vi "Get Timestamp s.vi"(9 "error in":errorcluster) -> (1 "error out":errorcluster, 2 "Timestamp":u64 format="%d ms")   [LabVIEW 2025, in "NET based Helpers.lvlib"]
uses:
  NET based Helpers.lvlib
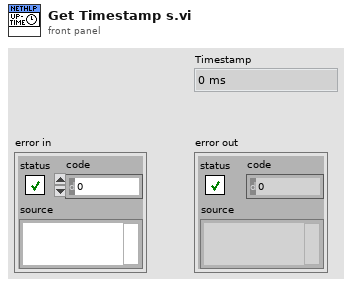
[diagram p1: front panel]
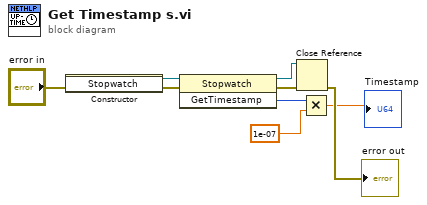
[diagram p0: block diagram]
diagram:
  n1 = constructor class="Stopwatch"(error in="error in") -> (reference out=w8:refnum<k24>, error out=w6:errorcluster)  [unwired: 2 in, 1 out]
  n2 = invoke class="Stopwatch" method="GetTimestamp"(reference=w8, error in=w6) -> (reference out=w5:refnum<k24>, error out=w4:errorcluster, "GetTimestamp"=w7:i64)  [unwired: 1 in]
  n3 = Close Reference(reference=w5, error in (no error)=w4) -> (error out=→"error out":errorcluster)
  n4 = Multiply(x=w7, y=1e-07) -> (x*y=→"Timestamp":dbl)
